vi "swag 2.vi"(1 "Numeric":dbl) -> (0 "°Farenheit":dbl(slide) scale=-100.0..300.0)   [LabVIEW 2014]
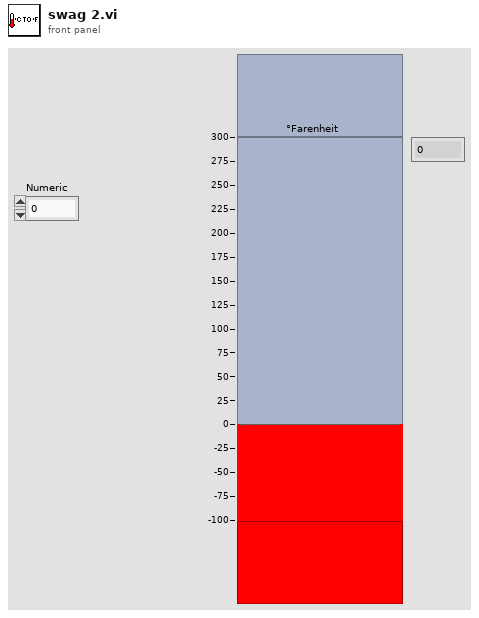
[diagram p1: front panel]
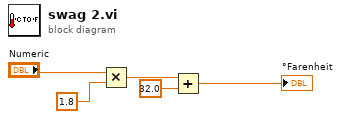
[diagram p0: block diagram]
diagram:
  n1 = Multiply(x="Numeric", y=1.8) -> (x*y=w3:dbl)
  n2 = Add(x=w3, y=32.0) -> (x+y=→"°Farenheit":dbl)
